vi "Read_Write_Local_table.vi"(3 "Mode":T8, 4 "Ch Values in":T1[](array[typedef]) {"New Value" format="%.2f"}, 5 "Channels Descriptions In":T2[](array[typedef]) {"Duty" format="%.0b"; "D" format="%#_5g"; "C" format="%#_5g"; "B" format="%#_5g"; "A" format="%#_5g"}) -> (0 "Ch Names":string[](array[string]), 1 "Ch Values Out":T1[](array[typedef]) {"New Value" format="%.2f"}, 2 "Channels Descriptions Out":T2[](array[typedef]) {"Duty" format="%.0b"; "D" format="%#_5g"; "C" format="%#_5g"; "B" format="%#_5g"; "A" format="%#_5g"})   [LabVIEW 2013]
uses:
  Anemometry/Anemometry Sub Vis/Controls/Global_mode.ctl
  ADAM Controls/Ch_description_ADAM.ctl
  ADAM Controls/Module_type_ADAM.ctl
  ADAM Controls/Function_ADAM.ctl
  ADAM Controls/Channel_State.ctl
  ADAM Controls/Calib_type_ADAM.ctl
  ADAM Controls/Address.ctl
  ADAM Controls/Update_scan_value.ctl
  Anemometry/Anemometry Sub Vis/Globals/Constants_global.vi
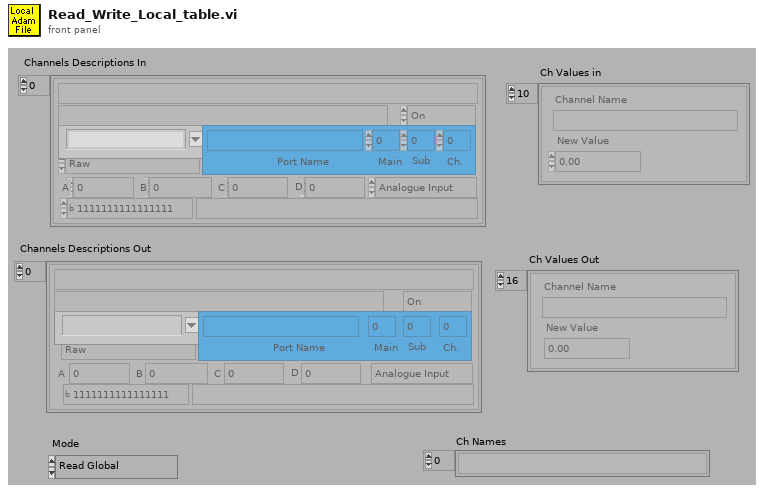
[diagram p1: front panel]
types:
  T1 = typedef "Update_scan_value.ctl" = cluster{"Channel Name":string, "New Value":dbl}
  T2 = typedef "Ch_description_ADAM.ctl" = cluster{"Ch Name":string, "Type":T3, "Function":T4, "Ch State":T5, "Calibration type":T6, "A":dbl, "B":dbl, "C":dbl, "D":dbl, "Comments":string, "Address":T7, "String":string, "Duty":u16}
  T3 = typedef "Module_type_ADAM.ctl" = string
  T4 = typedef "Function_ADAM.ctl" = enum16{"Analogue Input", "Digital Input", "Event counter", "Event rate", "Analogue Output", "Digital Output", "Relay Output"}
  T5 = typedef "Channel_State.ctl" = enum16{"On", "Off", "Always On", "Always Off"}
  T6 = typedef "Calib_type_ADAM.ctl" = enum16{"Raw", "Bx + A", "Cx^2 + Bx + A", "Dx^3 + Cx^2 + Bx + A", "In Band", "Hi-Tec Q", "Hi-Tec M_dot", "Text"}
  T7 = typedef "Address.ctl" = cluster{"Main":i32, "Ch.":i32, "Sub":i32, "Port Name":string}
  T8 = typedef "Global_mode.ctl" = enum16{"Read Global", "Load Global From File", "Write Global to File"}
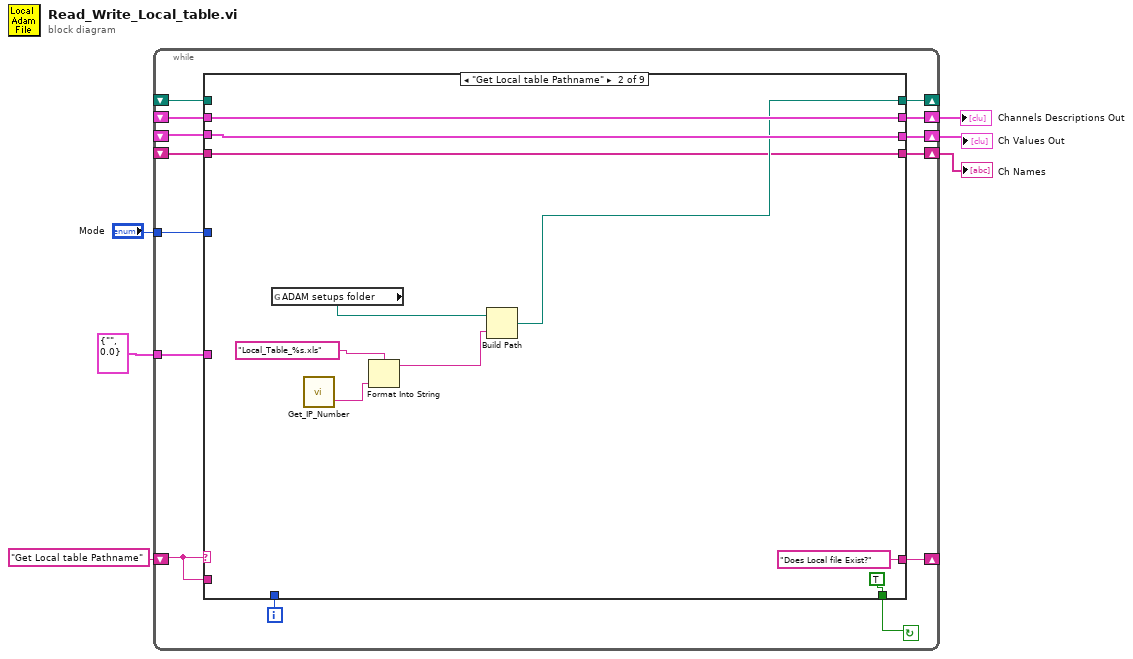
[diagram p0: block diagram]
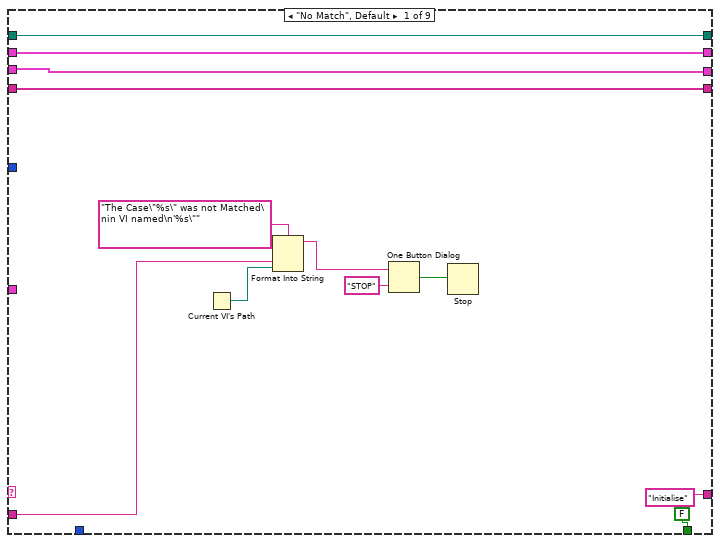
[diagram p2: hidden frame]
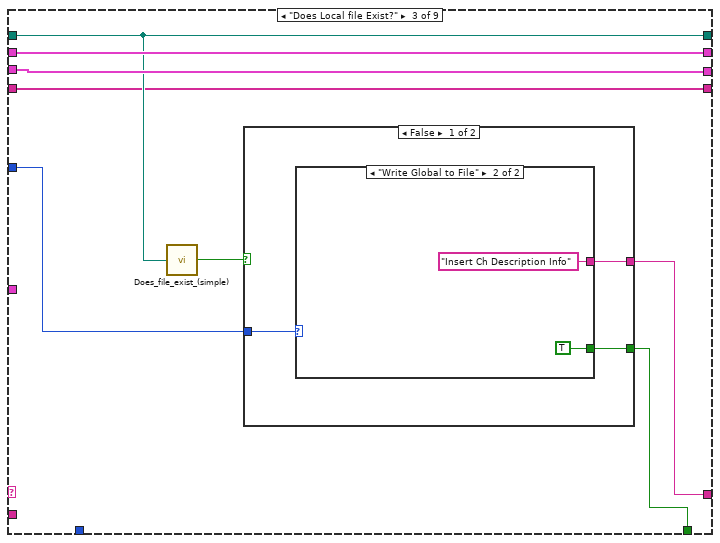
[diagram p3: hidden frame]
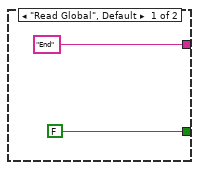
[diagram p4: hidden frame]
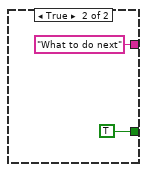
[diagram p5: hidden frame]
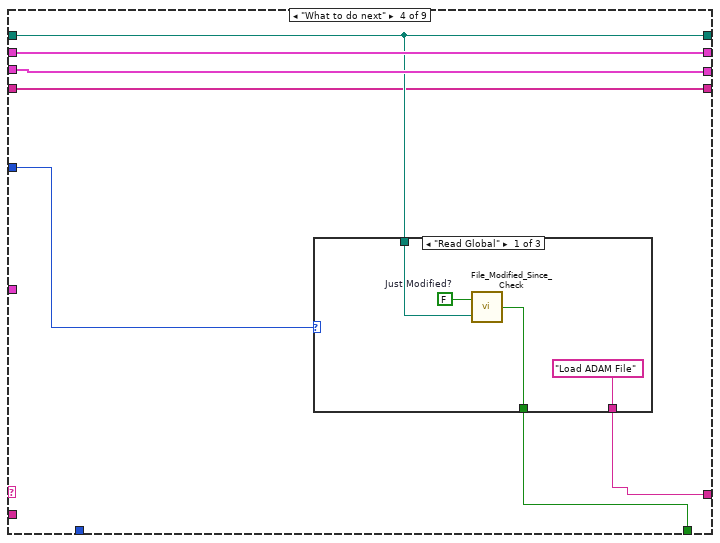
[diagram p6: hidden frame]
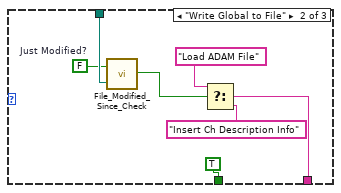
[diagram p7: hidden frame]
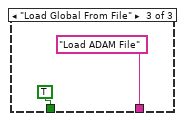
[diagram p8: hidden frame]
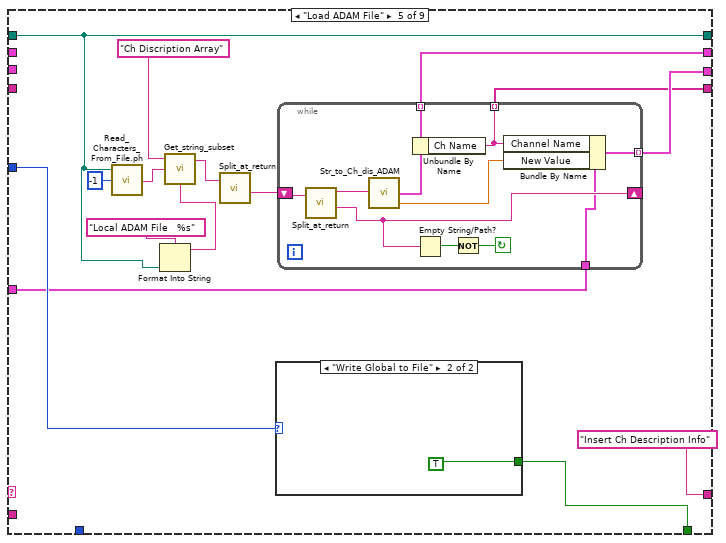
[diagram p9: hidden frame]
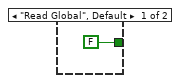
[diagram p10: hidden frame]
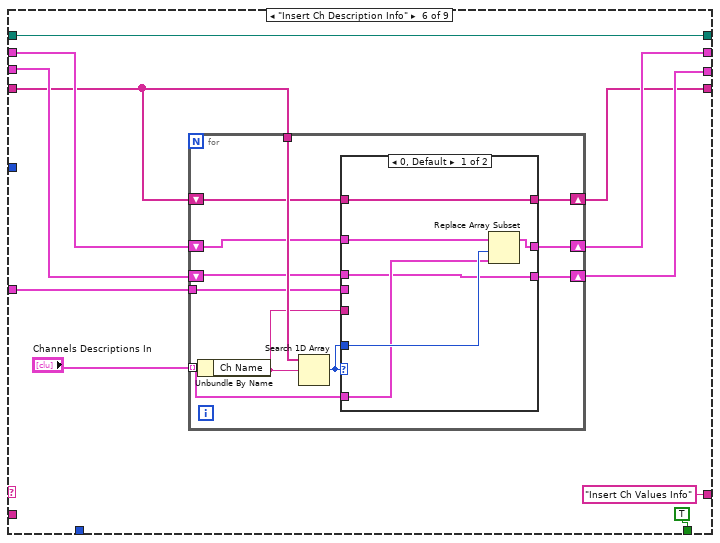
[diagram p11: hidden frame]
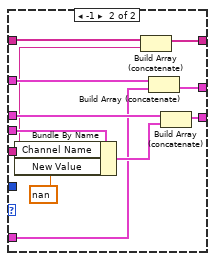
[diagram p12: hidden frame]
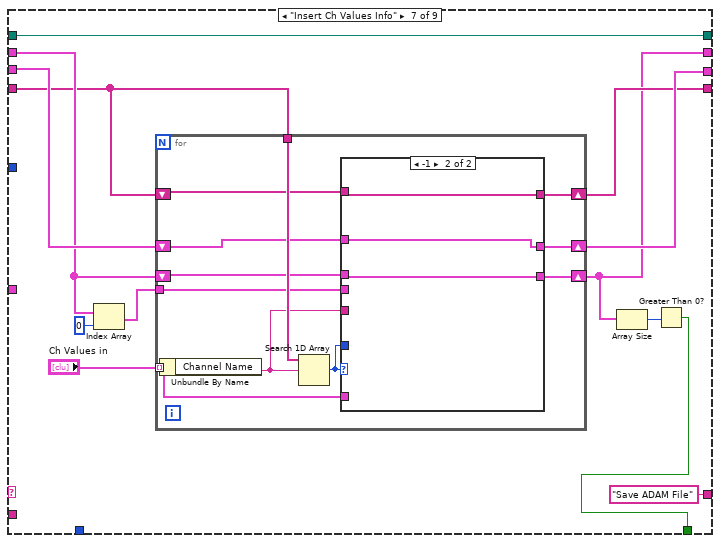
[diagram p13: hidden frame]
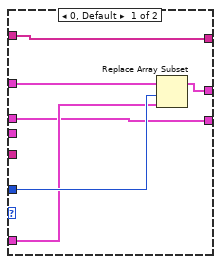
[diagram p14: hidden frame]
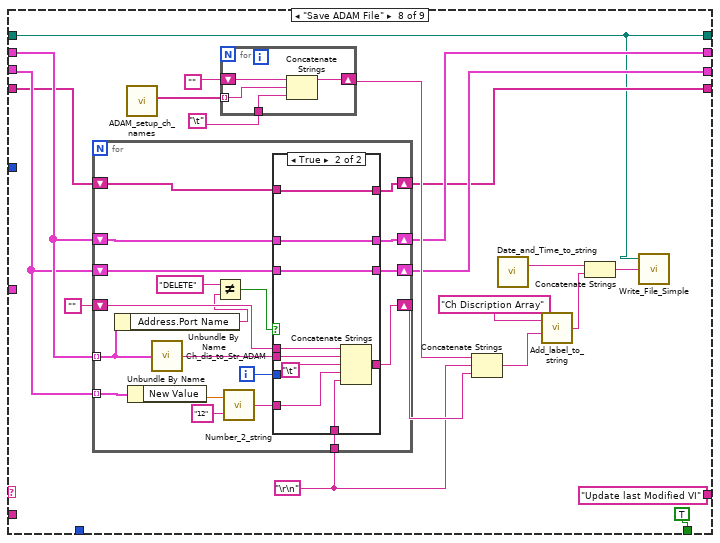
[diagram p15: hidden frame]
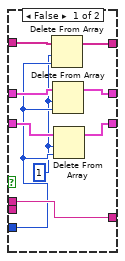
[diagram p16: hidden frame]
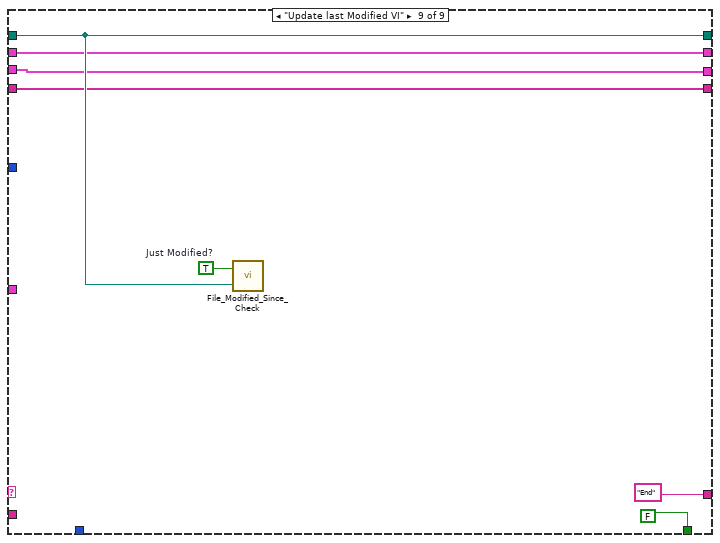
[diagram p17: hidden frame]
diagram:
  n1 = while {
    shift-left: _ -> [w7]
    shift-right: [w8] -> w1
    tunnel: T1 {"Channel Name"="", "New Value"=0.0} ("Update Scan Value Cluster") -> [w9]
    shift-left: _ -> [w11]
    shift-right: [w12] -> w2
    shift-left: _ -> [w13]
    shift-right: [w14] -> w4
    shift-left: _ -> [w17]
    shift-right: [w16] -> _
    tunnel: "Mode" -> [w18]
    shift-left: "Get Local table Pathname" -> [w15]
    shift-right: [w19] -> _
    i -> [w10]
    stop <- w20 continue-if-true
    n2 = case shown="\"Get Local table Pathname\"" w15 {
      tunnel: [FALSE TRUE w45 w63 w86 TRUE ("Modified?") w146 TRUE FALSE] -> w20
      tunnel: ["Initialise" "Does Local file Exist?" w46 w60 "Insert Ch Description Info" "Insert Ch Values Info" "Save ADAM File" "Update last Modified VI" "End"] -> w19
      tunnel: w18 -> [_ _ w47 w64 w87 _ _ _ _]
      tunnel: w17 -> [w25 _ w44 w62 w81 w109 w157 w181 w246]
      tunnel: [w25 w38 w44 w62 w81 w109 w157 w181 w246] -> w16
      tunnel: w15 -> [w27 _ _ _ _ _ _ _ _]
      tunnel: [w26 w41 w50 w66 w88 w114 w148 w184 w245] -> w14
      tunnel: w13 -> [w26 w41 w50 w66 _ w116 w153 w187 w245]
      tunnel: [w22 w40 w49 w65 w84 w113 w152 w185 w243] -> w12
      tunnel: w11 -> [w22 w40 w49 w65 _ w115 w154 w186 w243]
      tunnel: w10 -> [_ _ _ _ _ _ _ _ _]
      tunnel: w9 -> [_ _ _ _ w85 w112 _ _ _]
      tunnel: [w21 w36 w43 w61 w83 w107 w149 w182 w242] -> w8
      tunnel: w7 -> [w21 w36 w43 w61 _ w108 w150 w183 w242]
      frame "No Match", Default {
        n3 = Current VI's Path() -> (path=w28:path)
        n4 = Format Into String(format string="The Case\"%s\" was not Matched\nin VI named\n'%s\"" ("Format String"), w27, w28) -> (resulting string=w31:string)  [unwired: 2 in, 1 out]
        n5 = One Button Dialog(message=w31, button name ("OK")="STOP") -> (true=w29:bool)
        n6 = Stop(stop? (T)=w29) -> ()
      }
      frame "Get Local table Pathname" {
        n7 = global read "Constants_global.vi" "ADAM setups folder"() -> (w39:path)
        n8 = call "Get_IP_Number.vi"() -> ("Computer Name"=w34:string)  [unwired: 1 out]
        n9 = Format Into String(format string="Local_Table_%s.xls" ("name or relative path"), w34) -> (resulting string=w33:string)  [unwired: 2 in, 1 out]
        n10 = Build Path(base path=w39, name or relative path=w33) -> (appended path=w38:path)
      }
      frame "Does Local file Exist?" {
        n11 = call "Does_file_exist_(simple).vi"("Pathname"=w44) -> ("exists?"=w48:bool)
        n12 = case shown="False" w48 {
          tunnel: w47 -> [w53 _]
          tunnel: [w52 "What to do next"] -> w46
          tunnel: [w51 TRUE] -> w45
          frame False {
            n13 = case shown="\"Write Global to File\"" w53 {
              tunnel: ["End" "Insert Ch Description Info"] -> w52
              tunnel: [FALSE TRUE] -> w51
              frame "Read Global", Default {
              }
              frame "Write Global to File" {
              }
            }
          }
          frame True {
          }
        }
      }
      frame "What to do next" {
        n14 = case shown="\"Read Global\"" w64 {
          tunnel: w62 -> [w70 w77 _]
          tunnel: [w69 TRUE ("Modified?") TRUE ("Modified?")] -> w63
          tunnel: ["Load ADAM File" w72 "Load ADAM File"] -> w60
          frame "Read Global" {
            w67 = FALSE  # Just Modified?
            n15 = call "File_Modified_Since_Check.vi"("Pathname"=w70, "Just Modified?"=w67) -> ("Modified?"=w69:bool)
          }
          frame "Write Global to File" {
            w71 = FALSE  # Just Modified?
            n16 = call "File_Modified_Since_Check.vi"("Pathname"=w77, "Just Modified?"=w71) -> ("Modified?"=w76:bool)
            n17 = Select(t="Load ADAM File", s=w76, f="Insert Ch Description Info") -> (s? t:f=w72:string)
          }
          frame "Load Global From File" {
          }
        }
      }
      frame "Load ADAM File" {
        n18 = call "Read_Characters_From_File.ph.vi"("file path (dialog if empty)"=w81, "number of characters (all:-1)"=-1) -> ("character string"=w89:string)  [unwired: 7 out]
        n19 = Format Into String(format string="Local ADAM File   %s", w81) -> (resulting string=w80:string)  [unwired: 2 in, 1 out]
        n20 = call "Get_string_subset.vi"("String Name"=w80, "String to split"=w89, "File Label"="Ch Discription Array") -> ("Output string"=w91:string)  [unwired: 1 in, 1 out]
        n21 = call "Split_at_return.vi"("String"=w91) -> ("after substring"=w90:string)  [unwired: 1 in, 3 out]
        n22 = case shown="\"Write Global to File\"" w87 {
          tunnel: [FALSE TRUE] -> w86
          frame "Read Global", Default {
          }
          frame "Write Global to File" {
          }
        }
        n23 = while {
          tunnel: [w95] -> w83 mode=indexing
          tunnel: [w97] -> w84 mode=indexing
          tunnel: w85 -> [w99]
          tunnel: [w100] -> w88 mode=indexing
          shift-left: w90 -> [w104]
          shift-right: [w102] -> _
          stop <- w101 continue-if-true
          n24 = call "Split_at_return.vi"("String"=w104) -> ("before substring"=w103:string, "after substring"=w102:string)  [unwired: 1 in, 2 out]
          n25 = call "Str_to_Ch_dis_ADAM.vi"("String Row"=w103) -> ("Value"=w98:dbl, "Ch Description"=w100:T2)  [unwired: 1 in, 2 out]
          n26 = Unbundle By Name(w100) -> ("Ch Name"=w95:string)
          n27 = Empty String/Path?(string/path=w102) -> (empty?=w96:bool)
          n28 = Not(x=w96) -> (.not. x?=w101:bool)
          n29 = Bundle By Name(cluster=w99, "Channel Name"=w95, "New Value"=w98) -> (w97:T1)
        }
      }
      frame "Insert Ch Description Info" {
        n30 = for {
          tunnel: "Channels Descriptions In" -> [w121] mode=indexing
          tunnel: w108 -> [w128]
          shift-right: [w125] -> w114
          shift-left: w116 -> [w126]
          shift-right: [w124] -> w113
          shift-left: w115 -> [w127]
          tunnel: w112 -> [w123]
          shift-right: [w119] -> w107
          shift-left: w108 -> [w118]
          n31 = Unbundle By Name(w121) -> ("Ch Name"=w122:string)
          n32 = Search 1D Array(1D array=w128, element=w122) -> (index of element=w120:i32)  [unwired: 1 out]
          n33 = case shown="0, Default" w120 {
            tunnel: w127 -> [w130 w142]
            tunnel: w126 -> [w134 w145]
            tunnel: [w133 w144] -> w125
            tunnel: [w130 w143] -> w124
            tunnel: w123 -> [_ w141]
            tunnel: w122 -> [_ w135]
            tunnel: w121 -> [w131 w138]
            tunnel: w120 -> [w132 _]
            tunnel: [w129 w136] -> w119
            tunnel: w118 -> [w129 w137]
            frame 0, Default {
              n34 = Replace Array Subset(array=w134, new element=w131, index=w132) -> (w133:T2[])
            }
            frame -1 {
              n35 = Bundle By Name(cluster=w141, "Channel Name"=w135, "New Value"=nan ("Bundle Element")) -> (w140:T1)
              n36 = Build Array (concatenate)(w137, w135) -> (w136:string[])
              n37 = Build Array (concatenate)(w145, w138) -> (w144:T2[])
              n38 = Build Array (concatenate)(w142, w140) -> (w143:T1[])
            }
          }
        }
      }
      frame "Insert Ch Values Info" {
        n39 = Index Array(array=w153, index=0 ("Index")) -> (element=w151:T2)
        n40 = for {
          tunnel: "Ch Values in" -> [w162] mode=indexing
          tunnel: w150 -> [w169]
          shift-right: [w166] -> w152
          shift-left: w154 -> [w167]
          shift-right: [w165] -> w148
          shift-left: w153 -> [w168]
          tunnel: w151 -> [w164]
          shift-right: [w159] -> w149
          shift-left: w150 -> [w160]
          n41 = Unbundle By Name(w162) -> ("Channel Name"=w163:string)
          n42 = Search 1D Array(1D array=w169, element=w163) -> (index of element=w161:i32)  [unwired: 1 out]
          n43 = case shown="-1" w161 {
            tunnel: w168 -> [w171 w176]
            tunnel: w167 -> [w175 w177]
            tunnel: [w174 w177] -> w166
            tunnel: [w171 w176] -> w165
            tunnel: w164 -> [_ _]
            tunnel: w163 -> [_ _]
            tunnel: w162 -> [w172 _]
            tunnel: w161 -> [w173 _]
            tunnel: w160 -> [w170 w178]
            tunnel: [w170 w178] -> w159
            frame 0, Default {
              n44 = Replace Array Subset(array=w175, new element=w172, index=w173) -> (w174:T1[])
            }
            frame -1 {
            }
          }
        }
        n45 = Array Size(array=w148) -> (size(s)=w147:i32)
        n46 = Greater Than 0?(x=w147) -> (x > 0?=w146:bool)
      }
      frame "Save ADAM File" {
        w179 = "\r\n"
        n47 = for {
          tunnel: w187 -> [w215] mode=indexing
          shift-right: [w219] -> w189
          shift-left: "" -> [w220]
          tunnel: w186 -> [w218] mode=indexing
          shift-right: [w208] -> w185
          shift-left: w186 -> [w209]
          shift-right: [w210] -> w184
          shift-left: w187 -> [w211]
          shift-right: [w205] -> w182
          shift-left: w183 -> [w206]
          tunnel: w179 -> [w204]
          i -> [w207]
          n48 = Unbundle By Name(w215) -> ("Address.Port Name"=w214:string)
          n49 = Unbundle By Name(w218) -> ("New Value"=w217:dbl)
          n50 = call "Ch_dis_to_Str_ADAM.vi"("Ch Description"=w215) -> ("String Row"=w222:string)  [unwired: 4 out]
          n51 = Not Equal?(x="DELETE", y=w214) -> (x != y?=w212:bool)
          n52 = call "Number_2_string.vi"("precision"="12", "number"=w217) -> ("String"=w221:string)
          n53 = case shown="True" w212 {
            tunnel: w222 -> [_ w239]
            tunnel: w221 -> [_ w238]
            tunnel: w220 -> [w231 w237]
            tunnel: [w231 w236] -> w219
            tunnel: w211 -> [w230 w235]
            tunnel: [w229 w235] -> w210
            tunnel: w209 -> [w228 w234]
            tunnel: [w227 w234] -> w208
            tunnel: w207 -> [w224 _]
            tunnel: w206 -> [w226 w233]
            tunnel: [w225 w233] -> w205
            tunnel: w204 -> [_ w232]
            frame False {
              w223 = 1 ("length")
              n54 = Delete From Array(array=w226, length=w223, index=w224) -> (array with subset deleted=w225:string[])  [unwired: 1 out]
              n55 = Delete From Array(array=w230, length=w223, index=w224) -> (array with subset deleted=w229:T2[])  [unwired: 1 out]
              n56 = Delete From Array(array=w228, length=w223, index=w224) -> (array with subset deleted=w227:T1[])  [unwired: 1 out]
            }
            frame True {
              n57 = Concatenate Strings(w237, w239, "\t", w238, w232) -> (w236:string)
            }
          }
        }
        n58 = call "ADAM_setup_ch_names.vi"() -> ("Ch Names"=w196:string[])  [unwired: 1 out]
        n59 = for {
          shift-right: [w200] -> w188
          shift-left: "" -> [w203]
          tunnel: "\t" -> [w201]
          tunnel: w196 -> [w202] mode=indexing
          n60 = Concatenate Strings(w203, w202, w201) -> (w200:string)
        }
        n61 = Concatenate Strings(w188, w179, w189) -> (w192:string)
        n62 = call "Date_and_Time_to_string.vi"() -> ("Date and time (spreadsheet)"=w191:string)
        n63 = call "Add_label_to_string.vi"("String to write"=w192, "File Label"="Ch Discription Array") -> ("Output string"=w190:string)
        n64 = Concatenate Strings(w191, w190) -> (w180:string)
        n65 = call "Write_File_Simple.vi"("character string"=w180, "file path"=w181) -> ()  [unwired: 1 in, 2 out]
      }
      frame "Update last Modified VI" {
        w241 = TRUE  # Just Modified?
        n66 = call "File_Modified_Since_Check.vi"("Pathname"=w246, "Just Modified?"=w241) -> ()  [unwired: 1 out]
      }
    }
  }
  "Channels Descriptions Out" <- w4
  "Ch Values Out" <- w2
  "Ch Names" <- w1
